vi "3.3.vi"() -> ()   [LabVIEW 2020]
panel:
  out "Elipse":cluster{"X":dbl, "Y":dbl}[](graph)
  in  "B":dbl
  in  "A":dbl
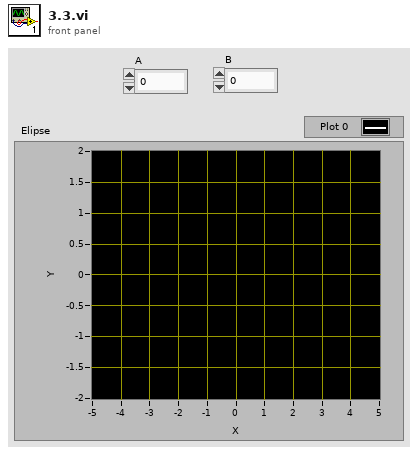
[diagram p1: front panel]
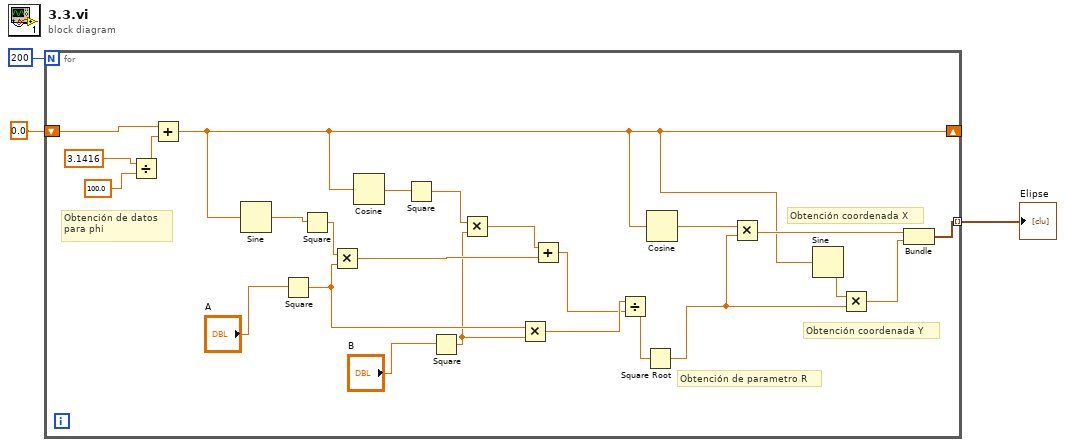
[diagram p0: block diagram]
diagram:
  n1 = for {
    N: 200 -> [_]
    shift-right: [w6] -> _
    shift-left: 0.0 -> [w27]
    tunnel: [w4] -> w1 mode=indexing
    # "Obtención coordenada Y"
    # "Obtención coordenada X"
    # "Obtención de parametro R"
    # "Obtención de datos \npara phi"
    n2 = Divide(x=3.1416 ("y"), y=100.0) -> (x/y=w24:dbl)
    n3 = Add(x=w27, y=w24) -> (x+y=w6:dbl)
    n4 = Sine(x=w6) -> (sin(x)=w23:dbl)
    n5 = Square(x="A") -> (x^2=w15:dbl)
    n6 = Square(x=w23) -> (x^2=w19:dbl)
    n7 = Multiply(x=w19, y=w15) -> (x*y=w16:dbl)
    n8 = Cosine(x=w6) -> (cos(x)=w22:dbl)
    n9 = Square(x=w22) -> (x^2=w18:dbl)
    n10 = Square(x="B") -> (x^2=w14:dbl)
    n11 = Multiply(x=w18, y=w14) -> (x*y=w17:dbl)
    n12 = Multiply(x=w15, y=w14) -> (x*y=w13:dbl)
    n13 = Add(x=w17, y=w16) -> (x+y=w12:dbl)
    n14 = Divide(x=w13, y=w12) -> (x/y=w11:dbl)
    n15 = Square Root(x=w11) -> (sqrt(x)=w8:dbl)
    n16 = Cosine(x=w6) -> (cos(x)=w10:dbl)
    n17 = Multiply(x=w10, y=w8) -> (x*y=w7:dbl)
    n18 = Sine(x=w6) -> (sin(x)=w9:dbl)
    n19 = Multiply(x=w9, y=w8) -> (x*y=w5:dbl)
    n20 = Bundle(w7, w5) -> (w4:cluster{dbl, dbl})  [unwired: 1 in]
  }
  "Elipse" <- w1
